vi "AAL Resample (const to variable, complex multi-channel).vi"(7 "reset? (True)":bool=TRUE, 8 "error in (no error)":errorcluster, 9 "config":T1={"timing jitter"=enum."Interpolation", "anti-aliasing?"=TRUE, "filter prototype"={"coefficients"=[], "factor"=1}} {"filter prototype"."coefficients" format="%.2f"}, 10 "time":dbl[](array[numeric]) format="%.2f", 11 "X":cdb[][](array[numeric])) -> (0 "error out":errorcluster, 1 "offset":i32, 2 "time stamps":dbl[](array[numeric]) format="%.2f", 3 "Y":cdb[][](array[numeric]) format="%.2f")   [LabVIEW 2010, in "NI_AALPro.lvlib"]
doc: "Perform an arbitrary resampling on the input signal."
uses:
  NI_AALPro.lvlib
  lvanlys.dll
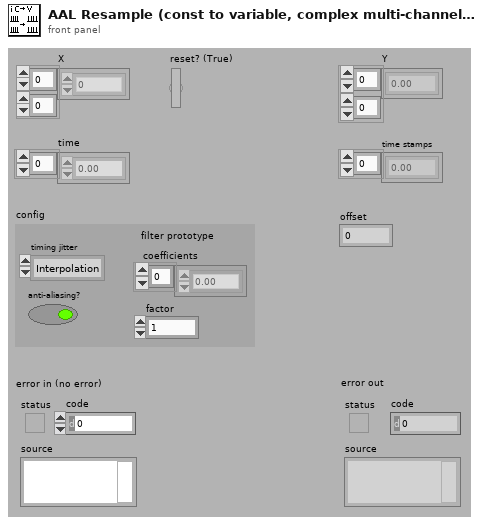
[diagram p1: front panel]
types:
  T1 = cluster{"timing jitter":enum32{"Interpolation", "Rounding"}, "anti-aliasing?":bool, "filter prototype":cluster{"coefficients":dbl[], "factor":i32}}
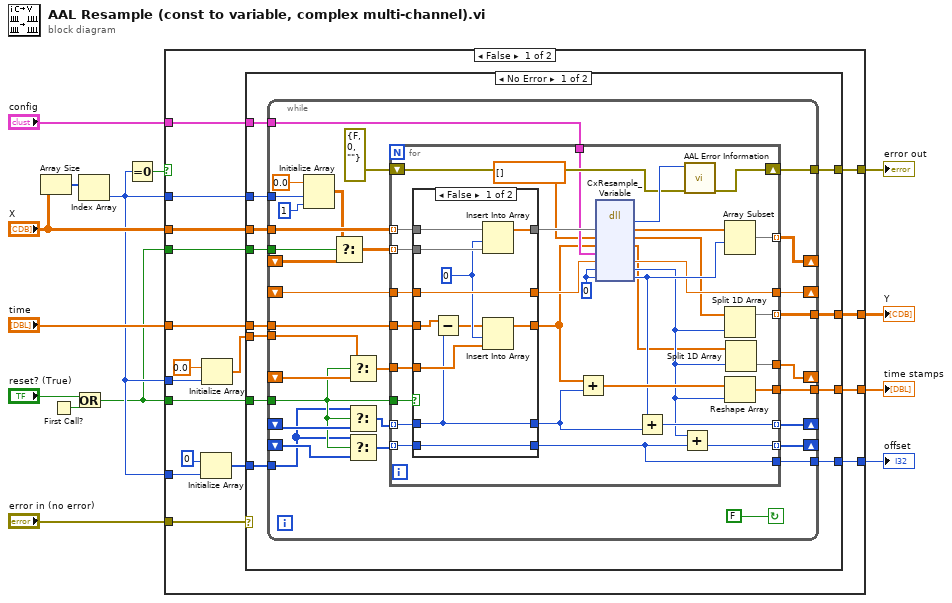
[diagram p0: block diagram]
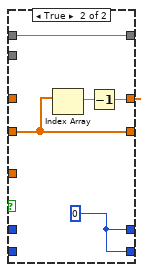
[diagram p2: hidden frame]
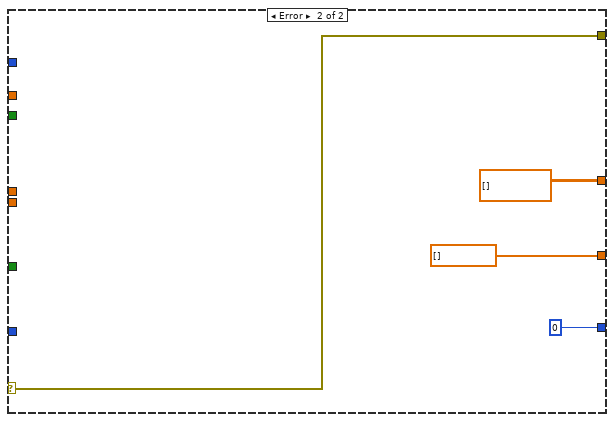
[diagram p3: hidden frame]
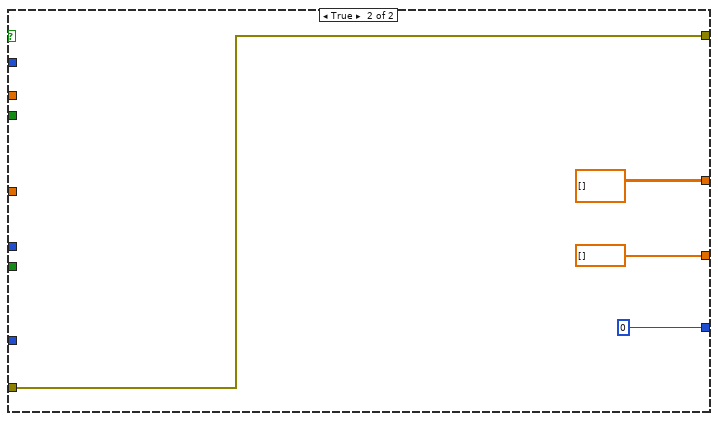
[diagram p4: hidden frame]
diagram:
  n1 = Array Size(array="X") -> (size(s)=w6:i32[])
  n2 = First Call?() -> (First Call?: T/F=w5:bool)
  n3 = Or(x="reset? (True)", y=w5) -> (x .or. y?=w1:bool)
  n4 = Index Array(array=w6) -> (element=w2:i32)  [unwired: 1 in]
  n5 = Equal To 0?(x=w2) -> (x = 0?=w3:bool)
  n6 = case shown="False" w3 {
    tunnel: "config" -> [w31 _]
    tunnel: "time" -> [w30 _]
    tunnel: [w29 dbl[] []] -> w12
    tunnel: [w28 dbl[][] []] -> w11
    tunnel: [w27 0 ("element")] -> w10
    tunnel: [w26 w128] -> w9
    tunnel: "error in (no error)" -> [w25 w128]
    tunnel: "X" -> [w24 _]
    tunnel: w1 -> [w21 _]
    tunnel: w2 -> [w19 _]
    tunnel: w2 -> [w17 _]
    tunnel: w2 -> [w16 _]
    tunnel: w1 -> [w15 _]
    frame False {
      n7 = Initialize Array(0 ("element"), w16) -> (w18:i32[])
      n8 = Initialize Array(0.0 ("element"), w17) -> (w20:dbl[])
      n9 = case shown="No Error" w25 {
        selector: w25 -> [_ w126]
        tunnel: w31 -> [w43 _]
        tunnel: w30 -> [w38 _]
        tunnel: [w42 dbl[] []] -> w29
        tunnel: [w41 cdb[][] []] -> w28
        tunnel: [w40 0] -> w27
        tunnel: [w39 w126] -> w26
        tunnel: w24 -> [w37 _]
        tunnel: w21 -> [w36 _]
        tunnel: w19 -> [w35 _]
        tunnel: w15 -> [w34 _]
        tunnel: w20 -> [w33 _]
        tunnel: w18 -> [w32 _]
        frame No Error {
          n10 = while {
            tunnel: [w66] -> w41
            tunnel: [w62] -> w42
            shift-right: [w72] -> _
            shift-left: _ -> [w52]
            shift-right: [w73] -> _
            shift-left: _ -> [w57]
            tunnel: w37 -> [w69]
            tunnel: w38 -> [w68]
            shift-right: [w71] -> _
            shift-left: _ -> [w67]
            tunnel: w36 -> [w45]
            tunnel: w43 -> [w74]
            shift-right: [w65] -> _
            shift-left: _ -> [w46]
            tunnel: [w64] -> w40
            shift-right: [w63] -> _
            shift-left: _ -> [w48]
            tunnel: [w60] -> w39
            tunnel: w34 -> [w58]
            tunnel: w35 -> [w53]
            tunnel: w33 -> [w50]
            tunnel: w32 -> [w44]
            stop <- FALSE continue-if-true
            n11 = Initialize Array(0.0, w53, 1 ("dimension size")) -> (w54:dbl[][])
            n12 = Select(t=w54, s=w58, f=w57) -> (s? t:f=w59:cdb[][])
            n13 = Select(t=w50, s=w45, f=w52) -> (s? t:f=w51:dbl[])
            n14 = Select(t=w44, s=w45, f=w46) -> (s? t:f=w47:i32[])
            n15 = Select(t=w44, s=w45, f=w48) -> (s? t:f=w49:i32[])
            n16 = for {
              tunnel: w74 -> [w81]
              tunnel: [w106] -> w73 mode=indexing
              tunnel: [w75] -> w72
              tunnel: [w83] -> w71
              tunnel: w69 -> [w105] mode=indexing
              tunnel: w68 -> [w103]
              tunnel: w59 -> [w102] mode=indexing
              tunnel: w51 -> [w101]
              tunnel: w67 -> [w100]
              tunnel: w45 -> [w99]
              tunnel: w47 -> [w98] mode=indexing
              tunnel: [w97] -> w66 mode=indexing
              tunnel: [w96] -> w65 mode=indexing
              tunnel: w49 -> [w93] mode=indexing
              tunnel: [w91] -> w64
              tunnel: [w90] -> w63 mode=indexing
              tunnel: [w88] -> w62
              shift-right: [w86] -> w60
              shift-left: errorcluster {"status"=FALSE, "code"=0, "source"=""} ("error out") -> [w87]
              w85 = 0
              n17 = case shown="False" w99 {
                tunnel: [w116 w122] -> w104
                tunnel: w105 -> [w114 w122]
                tunnel: [w111 w121] -> w79
                tunnel: w103 -> [w110 w121]
                tunnel: [w117 w119] -> w82
                tunnel: w102 -> [w113 _]
                tunnel: w101 -> [w115 _]
                tunnel: w100 -> [w117 _]
                tunnel: w98 -> [w108 _]
                tunnel: [w108 w118] -> w92
                tunnel: w93 -> [w107 _]
                tunnel: [w107 w118] -> w91
                frame False {
                  w112 = 0 ("Index")
                  n18 = Subtract(x=w110, y=w108) -> (x-y=w109:dbl[])
                  n19 = Insert Into Array(array=w114, index=w112, new element=w113) -> (w116:cdb[])
                  n20 = Insert Into Array(array=w109, index=w112, new element=w115) -> (w111:dbl[])
                }
                frame True {
                  w118 = 0
                  n21 = Index Array(array=w121) -> (element=w120:dbl)  [unwired: 1 in]
                  n22 = Decrement(x=w120) -> (x-1=w119:dbl)
                }
              }
              n23 = Add(x=w79, y=w92) -> (x+y=w95:dbl[])
              n24 = dll-call lib="C:/Program Files/National Instruments/LabVIEW 2010/resource/lvanlys.*" fn="CxResample_Variable"("X"=w104, "X"=cdb[] [], "timeH"=w79, "config"=w81, "last_sample_time"=w82, "out_len"=w85, "xLeftOverIdx"=w85) -> (w89:i32, "X"=w94:cdb[], "X"=w80:cdb[], "timeH"=w76:dbl[], "last_sample_time"=w83:dbl, "out_len"=w77:i32, "xLeftOverIdx"=w84:i32)  [unwired: 4 in, 2 out]
              n25 = Add(x=w84, y=w92) -> (x+y=w96:i32)
              n26 = Add(x=w77, y=w91) -> (x+y=w90:i32)
              n27 = call "AAL Error Information.vi"("error in (no error)"=w87, "error code"=w89) -> ("error out"=w86:errorcluster)  [unwired: 9 in]
              n28 = Array Subset(array=w94, index=w84) -> (w106:cdb[])  [unwired: 1 in]
              n29 = Split 1D Array(array=w80, index=w77) -> (first subarray=w97:cdb[])  [unwired: 1 out]
              n30 = Reshape Array(w95, w77) -> (w88:dbl[])
              n31 = Split 1D Array(array=w76, index=w77) -> (second subarray=w75:dbl[])  [unwired: 1 out]
            }
          }
        }
        frame Error {
        }
      }
    }
    frame True {
    }
  }
  "time stamps" <- w12
  "Y" <- w11
  "offset" <- w10
  "error out" <- w9
